vi "Ejercicio practica examen.vi"() -> ()   [LabVIEW 2011]
panel:
  out "mayor a 32":dbl
  out "rango 31-50":bool
  out "rango 21-30":bool
  out "rango 1-20":bool
  out "temp promedio":dbl
  out "temp mayor":dbl
  out "temp menor":dbl
  out "temperatura":i32(slide) scale=0.0..50.0
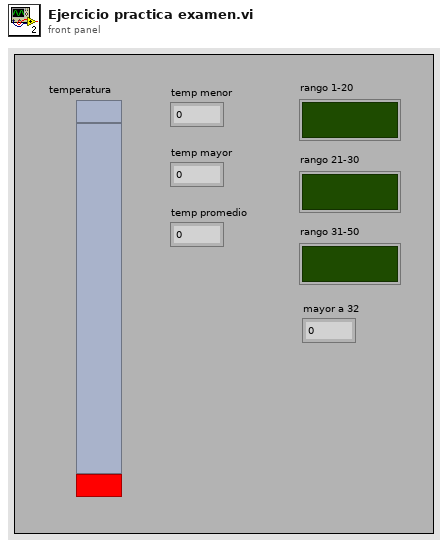
[diagram p1: front panel]
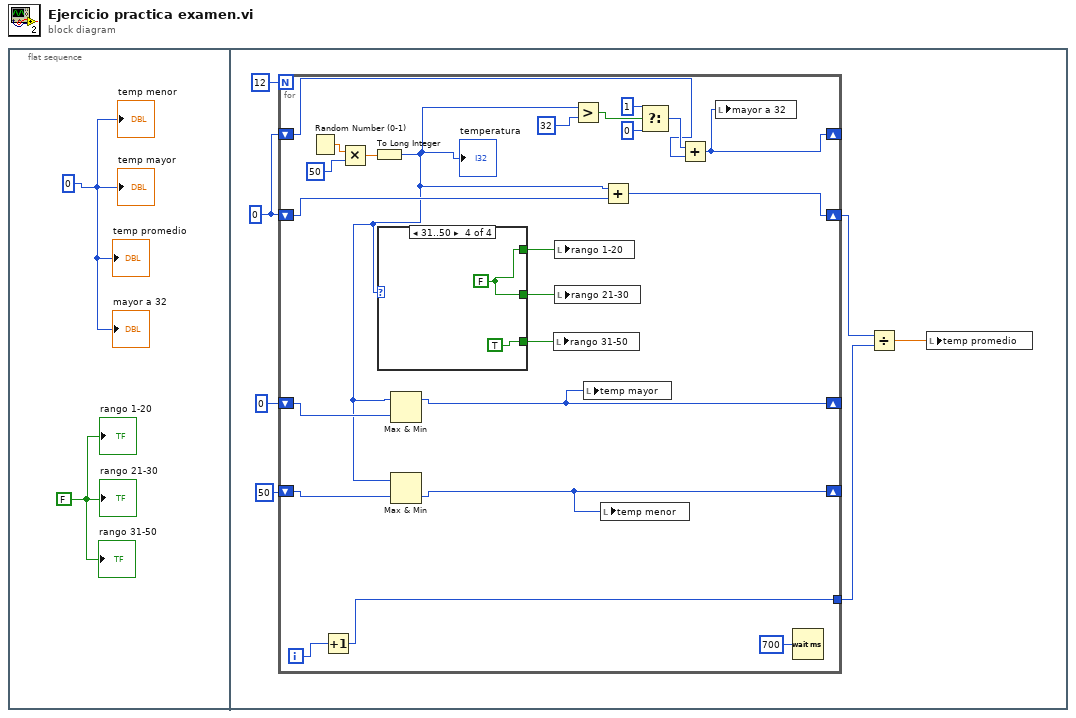
[diagram p0: block diagram]
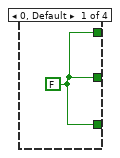
[diagram p2: hidden frame]
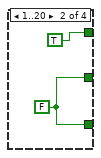
[diagram p3: hidden frame]
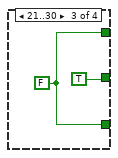
[diagram p4: hidden frame]
diagram:
  n1 = flat-sequence {
    frame #0 {
      w1 = FALSE
      w2 = 0
      "temp menor" <- w2
      "temp mayor" <- w2
      "temp promedio" <- w2
      "rango 1-20" <- w1
      "rango 21-30" <- w1
      "rango 31-50" <- w1
      "mayor a 32" <- w2
    }
    frame #1 {
      w3 = 0
      n2 = for {
        N: 12 -> [_]
        shift-right: [w20] -> _
        shift-left: 0 -> [w21]
        shift-right: [w18] -> _
        shift-left: 50 -> [w19]
        shift-right: [w15] -> w8
        shift-left: w3 -> [w17]
        tunnel: [w13] -> w7
        shift-right: [w10] -> _
        shift-left: w3 -> [w11]
        i -> [w14]
        n3 = Random Number (0-1)() -> (number: 0 to 1=w32:dbl)
        n4 = Increment(x=w14) -> (x+1=w13:i32)
        n5 = Multiply(x=w32, y=50) -> (x*y=w30:dbl)
        n6 = To Long Integer(number=w30) -> (32bit integer=w16:i32)
        "temperatura" <- w16
        n7 = case shown="31..50" w16 {
          tunnel: [w33 w34 TRUE w38] -> w29
          tunnel: [w33 w34 w36 TRUE] -> w28
          tunnel: [w33 TRUE w36 w38] -> w27
          frame 0, Default {
            w33 = FALSE
          }
          frame 1..20 {
            w34 = FALSE
          }
          frame 21..30 {
            w36 = FALSE
          }
          frame 31..50 {
            w38 = FALSE
          }
        }
        n8 = Max & Min(x=w16, y=w21) -> (max(x,y)=w20:i32)  [unwired: 1 out]
        n9 = Max & Min(x=w16, y=w19) -> (min(x,y)=w18:i32)  [unwired: 1 out]
        n10 = local write "rango 31-50"(w28) -> ()
        n11 = local write "rango 1-20"(w27) -> ()
        n12 = local write "rango 21-30"(w29) -> ()
        n13 = Greater?(x=w16, y=32) -> (0:w24:bool)
        n14 = local write "temp mayor"(w20) -> ()
        n15 = local write "temp menor"(w18) -> ()
        n16 = Add(x=w16, y=w17) -> (x+y=w15:i32)
        n17 = Select(t=1, s=w24, f=0) -> (s? t:f=w12:i32)
        n18 = Add(x=w12, y=w11) -> (x+y=w10:i32)
        n19 = local write "mayor a 32"(w10) -> ()
        n20 = Wait (ms)(milliseconds to wait=u32 700) -> ()  [unwired: 1 out]
      }
      n21 = Divide(x=w8, y=w7) -> (x/y=w6:dbl)
      n22 = local write "temp promedio"(w6) -> ()
    }
  }
